vi "input.vi"() -> ()   [LabVIEW 2015]
panel:
  out "String":string
  out "FG Data":T1
  in  "stop":bool
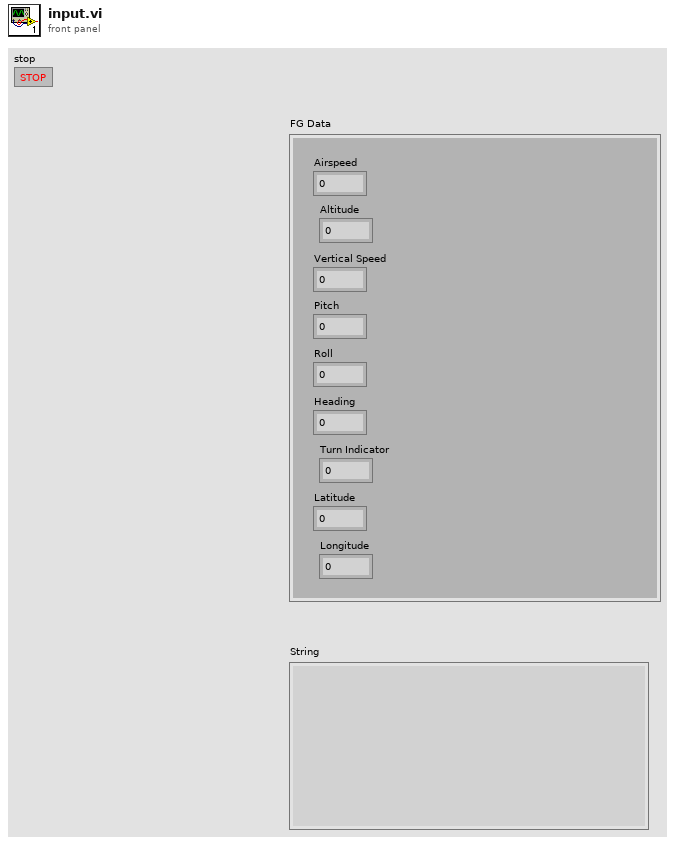
[diagram p1: front panel]
types:
  T1 = cluster{"Airspeed":dbl, "Altitude":dbl, "Vertical Speed":dbl, "Pitch":dbl, "Roll":dbl, "Heading":dbl, "Turn Indicator":dbl, "Latitude":dbl, "Longitude":dbl}
  T2 = cluster{dbl, dbl, dbl, dbl, dbl, dbl, dbl, dbl, dbl}
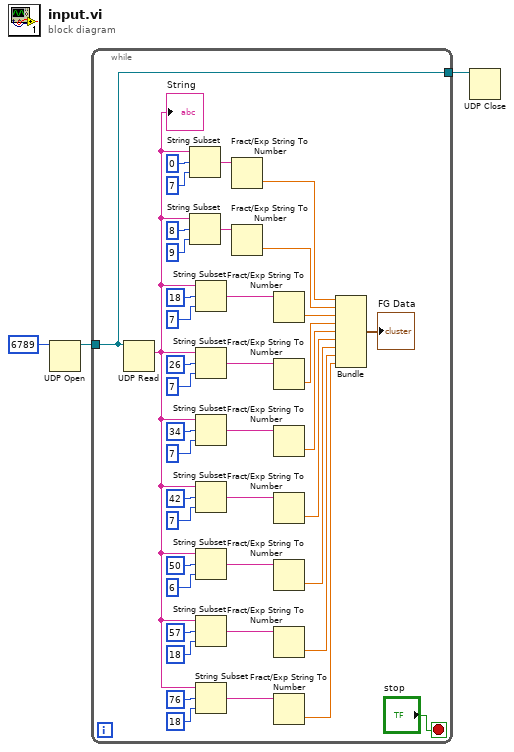
[diagram p0: block diagram]
diagram:
  n1 = UDP Open(11:u16 6789 ("port")) -> (port=w2:refnum<k16>)  [unwired: 4 in, 2 out]
  n2 = while {
    tunnel: w2 -> [w4]
    tunnel: [w4] -> w1
    stop <- "stop" stop-if-true
    n3 = UDP Read(connection ID=w4) -> (data out=w34:string)  [unwired: 3 in, 4 out]
    "String" <- w34
    n4 = String Subset(string=w34, offset (0)=0, length (rest)=7 ("length (rest)")) -> (substring=w5:string)
    n5 = String Subset(string=w34, offset (0)=8, length (rest)=9 ("length (rest)")) -> (substring=w37:string)
    n6 = String Subset(string=w34, offset (0)=18, length (rest)=7 ("length (rest)")) -> (substring=w33:string)
    n7 = String Subset(string=w34, offset (0)=26, length (rest)=7 ("length (rest)")) -> (substring=w32:string)
    n8 = String Subset(string=w34, offset (0)=34, length (rest)=7 ("length (rest)")) -> (substring=w31:string)
    n9 = String Subset(string=w34, offset (0)=42, length (rest)=7 ("length (rest)")) -> (substring=w30:string)
    n10 = String Subset(string=w34, offset (0)=50, length (rest)=6 ("length (rest)")) -> (substring=w29:string)
    n11 = String Subset(string=w34, offset (0)=57, length (rest)=18 ("length (rest)")) -> (substring=w28:string)
    n12 = String Subset(string=w34, offset (0)=76, length (rest)=18 ("length (rest)")) -> (substring=w27:string)
    n13 = Fract/Exp String To Number(string=w5) -> (number=w38:dbl)  [unwired: 3 in, 1 out]
    n14 = Fract/Exp String To Number(string=w37) -> (number=w36:dbl)  [unwired: 3 in, 1 out]
    n15 = Fract/Exp String To Number(string=w33) -> (number=w26:dbl)  [unwired: 3 in, 1 out]
    n16 = Fract/Exp String To Number(string=w32) -> (number=w25:dbl)  [unwired: 3 in, 1 out]
    n17 = Fract/Exp String To Number(string=w31) -> (number=w24:dbl)  [unwired: 3 in, 1 out]
    n18 = Fract/Exp String To Number(string=w30) -> (number=w23:dbl)  [unwired: 3 in, 1 out]
    n19 = Fract/Exp String To Number(string=w29) -> (number=w22:dbl)  [unwired: 3 in, 1 out]
    n20 = Fract/Exp String To Number(string=w28) -> (number=w21:dbl)  [unwired: 3 in, 1 out]
    n21 = Fract/Exp String To Number(string=w27) -> (number=w20:dbl)  [unwired: 3 in, 1 out]
    n22 = Bundle(w38, w36, w26, w25, w24, w23, w22, w21, w20) -> (→"FG Data":T2)  [unwired: 1 in]
  }
  n23 = UDP Close(connection ID=w1) -> ()  [unwired: 1 in, 2 out]
